vi "Camera test.vi"() -> ()   [LabVIEW 2020]
uses:
  <vilib>/userDefined/High Color/IMAQdx.ctl
panel:
  out "Session Out":T1
  in  "stop":bool
  out "Data":string
  out "Image":T2(plugin-control)
  in  "file (use dialog)":path
  in  "Session In":T1
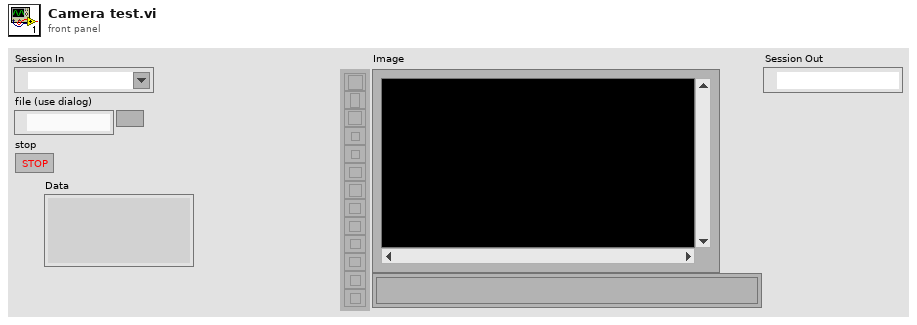
[diagram p1: front panel]
types:
  T1 = typedef "IMAQdx.ctl" = refnum<k21>
  T2 = typedef "IMAQ Image.ctl" = refnum<image>
  T3 = enum16{"open", "replace", "create", "open or create", "replace or create", "replace or create with confirmation"}
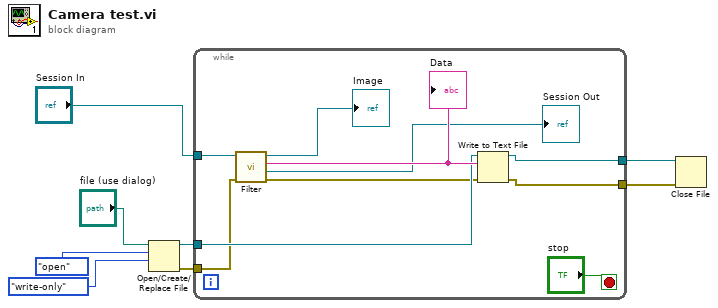
[diagram p0: block diagram]
diagram:
  n1 = Open/Create/Replace File(file path (use dialog)="file (use dialog)", operation (0:open)=T3."open", access (0:read/write)=enum16{"read/write", "read-only", "write-only"}."write-only") -> (refnum out=w3:refnum<file>, error out=w4:errorcluster)  [unwired: 3 in, 1 out]
  n2 = while {
    tunnel: "Session In" -> [w18]
    tunnel: w4 -> [w12]
    tunnel: w3 -> [w15]
    tunnel: [w14] -> w2
    tunnel: [w13] -> w1
    stop <- "stop" stop-if-true
    n3 = call "Filter.vi"("error in"=w12, "Session Config"=w18) -> ("error out"=w11:errorcluster, "Session Out"=→"Session Out":T1, "Data"=w17:string, "Image Out"=→"Image":T2)  [unwired: 6 in]
    "Data" <- w17
    n4 = Write to Text File(file (use dialog)=w15, text=w17, error in=w11) -> (refnum out=w13:refnum<file>, error out=w14:errorcluster)  [unwired: 1 in, 1 out]
  }
  n5 = Close File(refnum=w1, error in=w2) -> ()  [unwired: 2 out]
